vi "Agilent N6700 Series Configure Histogram.vi"() -> ()   [LabVIEW 2021]
doc: "Configure the histogram, histogram trigger source, initiates the histogram, triggers the histogram and fetches the histogram bin data.\n\n<b>Note:</b>\n\nThis VI only applies to the N6705B and N6705C DC Power Analyzer."
uses:
  <instrlib>/Agilent N6700 Series/Agilent N6700 Series.lvlib
panel:
  in  "error in":errorcluster {"code" format="%.0x"}
  out "error out":errorcluster {"code" format="%.0x"}
  in  "Wait Time":i32=1000
  out "Bin Data":dbl[](array[numeric]) format="%^.3e"
  in  "Histogram Trigger Source":i32(ring)=1 items=["External", "Software", "Immediate", "Pin 1", "Pin 2", "Pin 3"]
  in  "Histogram Range":dbl format="%^.3e"
  in  "Bin Range (0: 8 A)":i32(ring) items=["8 A", "0.0039 A"]
  in  "Channel Name":string="1"
  in  "Agilent SMU":refnum<visa-resource-name>
  # "(c) 2012-2019  National Instruments.  ALL RIGHTS RESERVED."
  # "Agilent N6705 DC Power Supply"
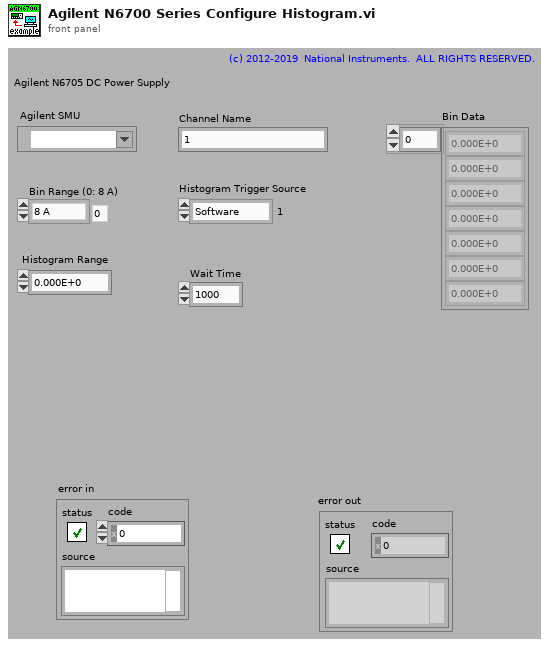
[diagram p1: front panel]
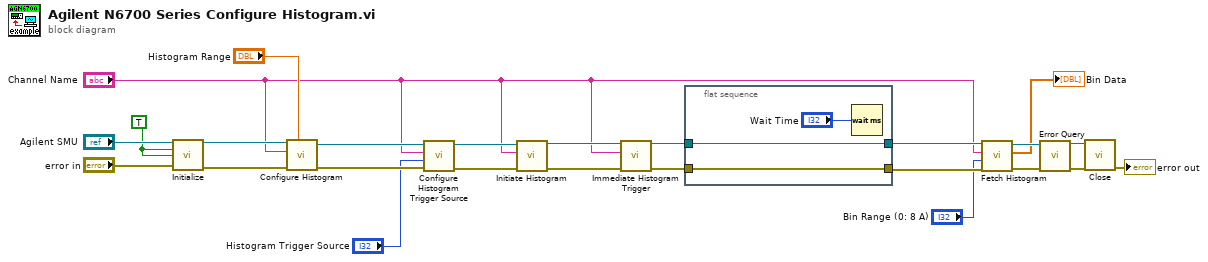
[diagram p0: block diagram]
diagram:
  w22 = TRUE ("Reset? (T: Yes)")
  n1 = call <instrlib>:"Initialize.vi"("VISA resource name"="Agilent SMU", "ID Query? (T: Yes)"=w22, "Reset? (T: Yes)"=w22, "error in (no error)"="error in") -> ("VISA resource name out"=w19:refnum<visa-resource-name>, "error out"=w18:errorcluster)  [unwired: 10 in]
  n2 = call <instrlib>:"Configure Histogram.vi"("Histogram Range (0.0)"="Histogram Range", "error in (no error)"=w18, "Channel Name (1)"="Channel Name", "VISA resource name"=w19) -> ("error out"=w17:errorcluster, "VISA resource name out"=w16:refnum<visa-resource-name>)  [unwired: 6 in]
  n3 = call <instrlib>:"Configure Histogram Trigger Source.vi"("error in (no error)"=w17, "Histogram Trigger Source (1: Software)"="Histogram Trigger Source", "Channel Name (1)"="Channel Name", "VISA resource name"=w16) -> ("error out"=w8:errorcluster, "VISA resource name out"=w9:refnum<visa-resource-name>)  [unwired: 6 in]
  n4 = call <instrlib>:"Initiate Histogram.vi"("error in (no error)"=w8, "Channel Name (1)"="Channel Name", "VISA resource name"=w9) -> ("error out"=w7:errorcluster, "VISA resource name out"=w10:refnum<visa-resource-name>)  [unwired: 7 in]
  n5 = call <instrlib>:"Immediate Histogram Trigger.vi"("error in (no error)"=w7, "Channel Name (1)"="Channel Name", "VISA resource name"=w10) -> ("error out"=w5:errorcluster, "VISA resource name out"=w6:refnum<visa-resource-name>)  [unwired: 7 in]
  n6 = flat-sequence {
    tunnel: w5 -> [w28]
    tunnel: [w28] -> w14
    tunnel: w6 -> [w27]
    tunnel: [w27] -> w15
    frame #0 {
      n7 = Wait (ms)(milliseconds to wait="Wait Time") -> ()  [unwired: 1 out]
    }
  }
  n8 = call <instrlib>:"Fetch Histogram.vi"("error in (no error)"=w14, "Bin Range (0: 8A)"="Bin Range (0: 8 A)", "Channel Name (1)"="Channel Name", "VISA resource name"=w15) -> ("error out"=w24:errorcluster, "Bin Data"=→"Bin Data":dbl[], "VISA resource name out"=w25:refnum<visa-resource-name>)  [unwired: 5 in]
  n9 = call <instrlib>:"Error Query.vi"("VISA resource name"=w25, "error in (no error)"=w24) -> ("VISA resource name out"=w20:refnum<visa-resource-name>, "error out"=w21:errorcluster)  [unwired: 10 in, 2 out]
  n10 = call <instrlib>:"Close.vi"("VISA resource name"=w20, "error in (no error)"=w21) -> ("error out"=→"error out":errorcluster)  [unwired: 13 in]
